vi "Initialize.vi"(8 "error in (no error)":errorcluster) -> (0 "error out":errorcluster)   [LabVIEW 2017, in "lvwpcap.lvlib"]
uses:
  lvwpcap.lvlib
  LVpcap.dll
panel:
  # "Select Help»Show Context Help and move the cursor over the VI icon to display help for this VI."
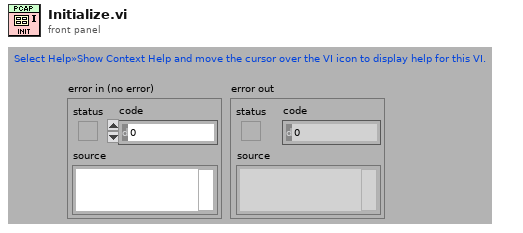
[diagram p1: front panel]
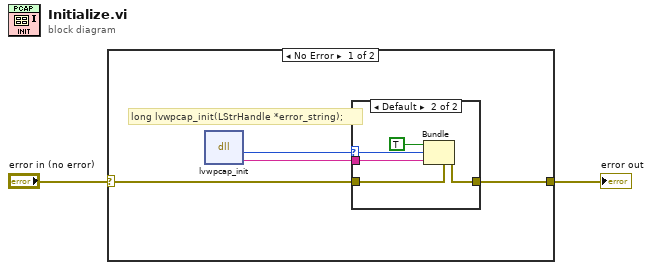
[diagram p0: block diagram]
diagram:
  n1 = case shown="No Error" "error in (no error)" {
    selector: "error in (no error)" -> [w3 w13]
    tunnel: [w4 w13] -> w2
    frame No Error {
      # "long lvwpcap_init(LStrHandle *error_string);"
      n2 = dll-call lib="C:/Users/Michaello/Desktop/MGR NOWEEEEEEEEEEEEEE/MR PROFINET 2017/Lib/WinPcap/LVpcap.dll" fn="lvwpcap_init"() -> ("return type"=w6:i32, "error_string"=w5:string)  [unwired: 4 in, 2 out]
      n3 = case shown="Default" w6 {
        selector: w6 -> [_ w11]
        tunnel: w5 -> [_ w10]
        tunnel: w3 -> [w7 w12]
        tunnel: [w7 w8] -> w4
        frame 0 {
        }
        frame Default {
          n4 = Bundle(cluster=w12, "status"=TRUE, "code"=w11, "source"=w10) -> (w8:errorcluster)
        }
      }
    }
    frame Error {
    }
  }
  "error out" <- w2
